vi "Array DBL поддержание размера.vi"(8 "Array size":i32=10, 10 "New element":dbl format="%#_13g", 11 "Array":dbl[](array[numeric])) -> (3 "Array out":dbl[](array[numeric]))   [LabVIEW 2023]
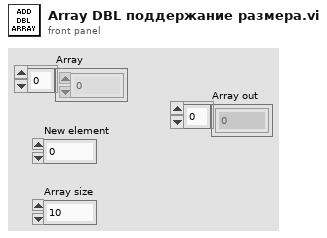
[diagram p1: front panel]
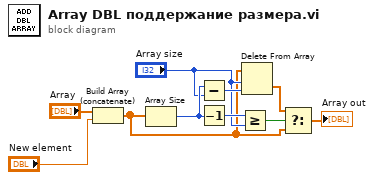
[diagram p0: block diagram]
diagram:
  n1 = Build Array (concatenate)("Array", "New element") -> (w3:dbl[])
  n2 = Array Size(array=w3) -> (size(s)=w8:i32)
  n3 = Subtract(x=w8, y="Array size") -> (x-y=w10:i32)
  n4 = Decrement(x=w8) -> (x-1=w9:i32)
  n5 = Greater Or Equal?(x=w9, y="Array size") -> (x >= y?=w2:bool)
  n6 = Delete From Array(array=w3, length="Array size", index=w10) -> (deleted portion=w4:dbl[])  [unwired: 1 out]
  n7 = Select(t=w4, s=w2, f=w3) -> (s? t:f=→"Array out":dbl[])
